vi "LS Durability Main ALTERNATE (FPGA).vi"() -> ()   [LabVIEW 2013]
uses:
  <vilib>/rvi/Emulation/niFpgaSctlEmulationGetInTimedLoop.vi
  <vilib>/rvi/Emulation/niFpgaEmulationReportErrorSimple.vi
  <vilib>/rvi/Emulation/niFpgaGetClockAttributes.vi
  <vilib>/rvi/eio/common/nirviEmuTemplateMethod_errors.vi
  <vilib>/rvi/Emulation/niFpgaCriticalErrorInLSC.vi
  <vilib>/eio/EIONode/EIONode.xnode
panel:
  out "Anomaly Resamples":fxp<+/-,28,17>[](array[numeric])
  in  "Anomaly Threshold":fxp<+/-,28,17>=0.02978515625
  out "Bank2Active":bool
  out "Bank1Active":bool
  out "Bank2On":bool
  out "Bank1On":bool
  in  "Enable Readings":bool[](array[boolean])=[FALSE, FALSE, FALSE, FALSE, FALSE, FALSE, FALSE, FALSE, FALSE, FALSE, FALSE, FALSE]
  in  "Opens Resets":bool[](array[boolean])=[FALSE, FALSE, FALSE, FALSE, FALSE, FALSE, FALSE, FALSE, FALSE, FALSE, FALSE, FALSE]
  in  "Enable Opens":bool[](array[boolean])=[FALSE, FALSE, FALSE, FALSE, FALSE, FALSE, FALSE, FALSE, FALSE, FALSE, FALSE, FALSE]
  out "Opens Detected":u16[](array[numeric])
  out "Opens Loop Time (usec)":u32=1000
  in  "Bank2(Pulse/Const)":bool
  in  "Bank2Const(On/Off)":bool
  out "Anomalies (Last Cycle)":i32[](array[numeric])
  out "Cycle Starts":bool[](array[boolean])
  out "Anomalies (Total)":i32[](array[numeric])
  out "Anomalies/Cycle":i32[](array[numeric])
  in  "Normal Steps":u32=98
  out "Cycles":u32[](array[numeric])
  out "Anomaly Loop Time (usec)":u32=1000
  out "Steps":u32[](array[numeric])
  in  "Step Threshold":fxp<+/-,28,17>=0.02978515625
  in  "Enable Anomalies":bool[](array[boolean])=[FALSE, FALSE, FALSE, FALSE, FALSE, FALSE, FALSE, FALSE, FALSE, FALSE, FALSE, FALSE]
  in  "Anomaly Resets":bool[](array[boolean])=[FALSE, FALSE, FALSE, FALSE, FALSE, FALSE, FALSE, FALSE, FALSE, FALSE, FALSE, FALSE]
  in  "Bank1Const(On/Off)":bool
  in  "Bank1(Pulse/Const)":bool
  in  "PWM Period (Ticks)":u32=4000000
  in  "Duty (Ticks)":i32=2000000
  in  "Invert PWM?":bool=TRUE
  in  "Cycle Resets":bool[](array[boolean])=[FALSE, FALSE, FALSE, FALSE, FALSE, FALSE, FALSE, FALSE, FALSE, FALSE, FALSE, FALSE]
  in  "Points to Avg":i32=20
  in  "Enable Cycles":bool[](array[boolean])=[FALSE, FALSE, FALSE, FALSE, FALSE, FALSE, FALSE, FALSE, FALSE, FALSE, FALSE, FALSE]
  out "Total Cycles":u32[](array[numeric])
  in  "Cycle Threshold":fxp<+/-,28,17>=1.2001953125
  out "AI Avg Loop Time (usec)":u32=1000
  out "Analog Inputs":fxp<+/-,28,17>[](array[numeric])
  out "AI Loop Time (usec)":u32=70
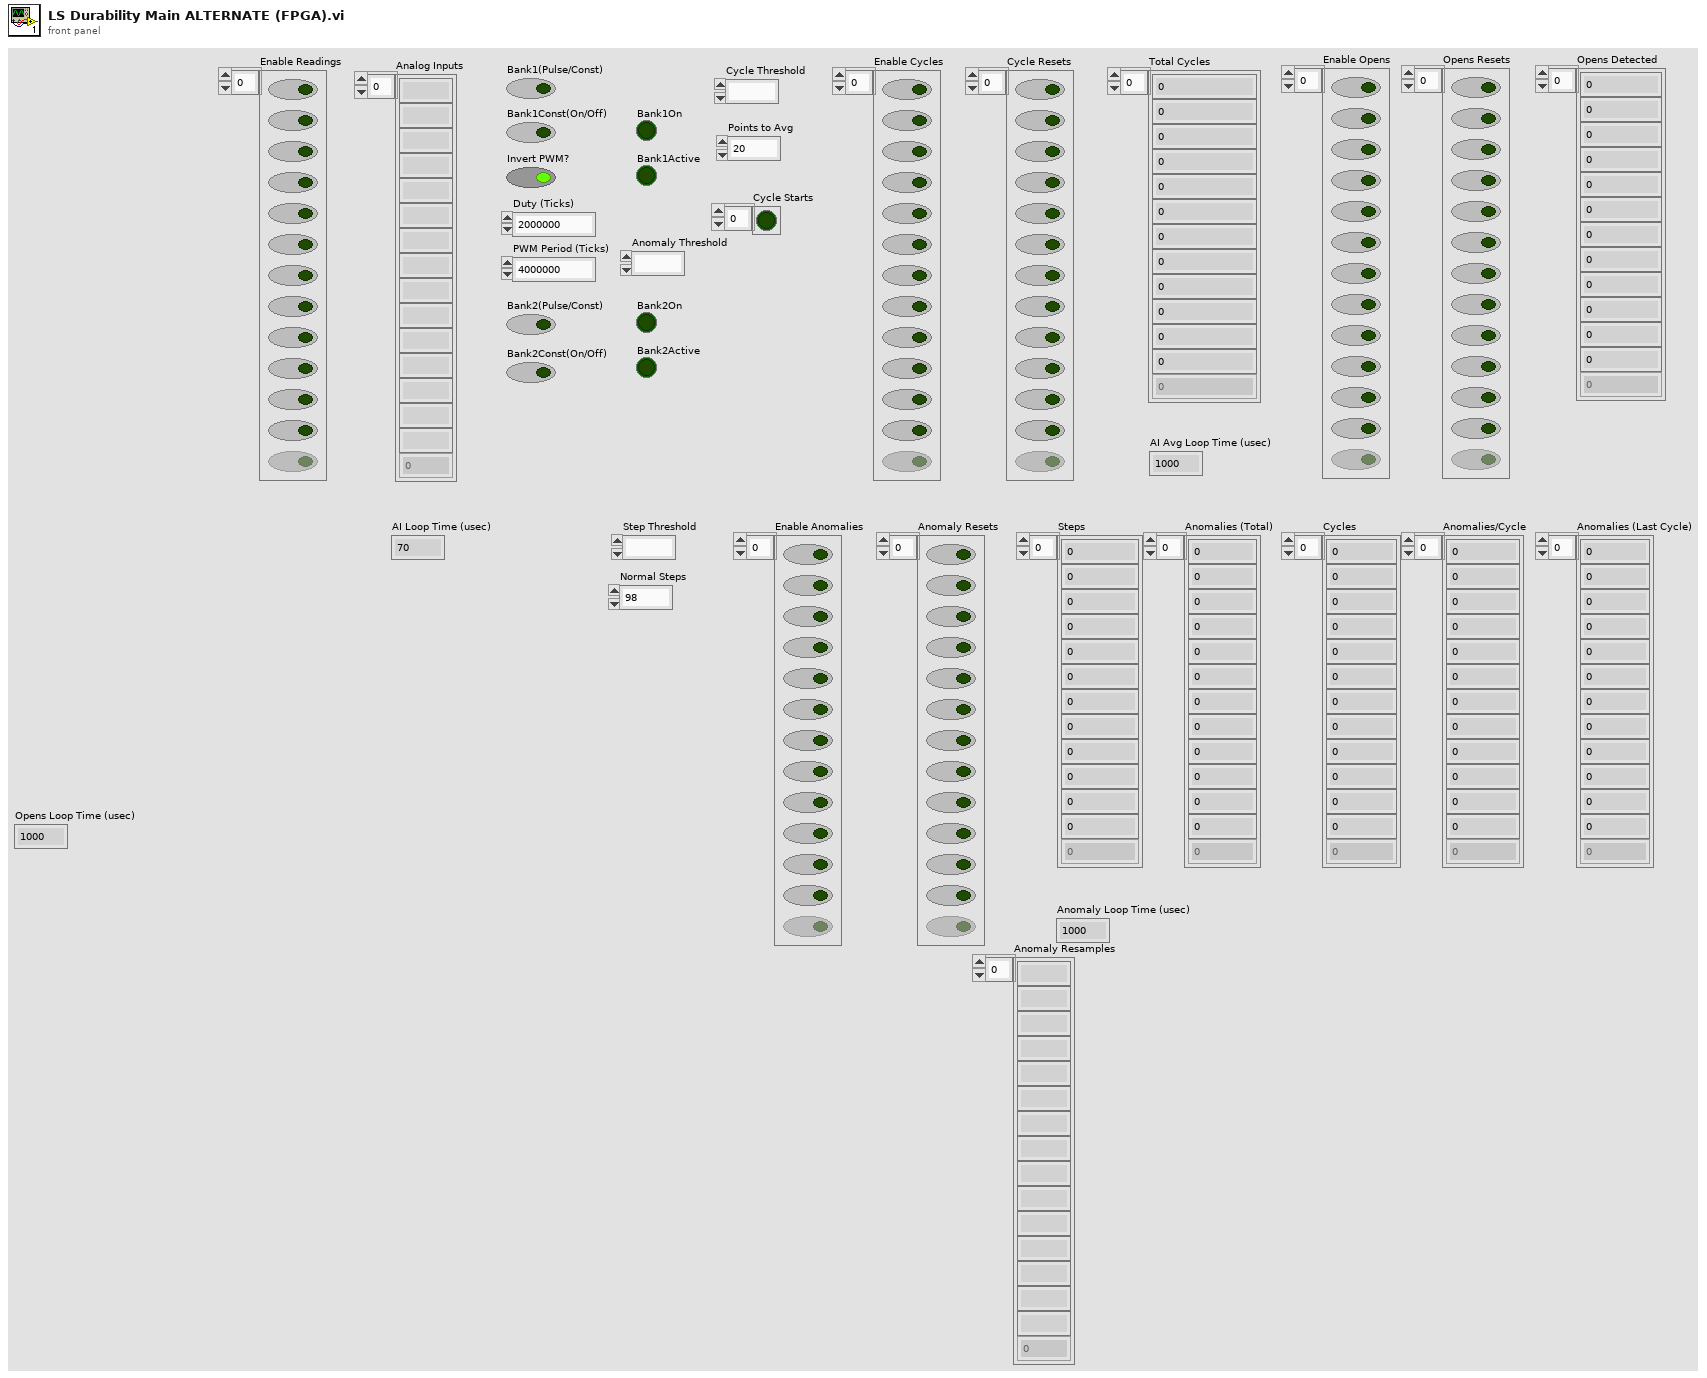
[diagram p1: front panel]
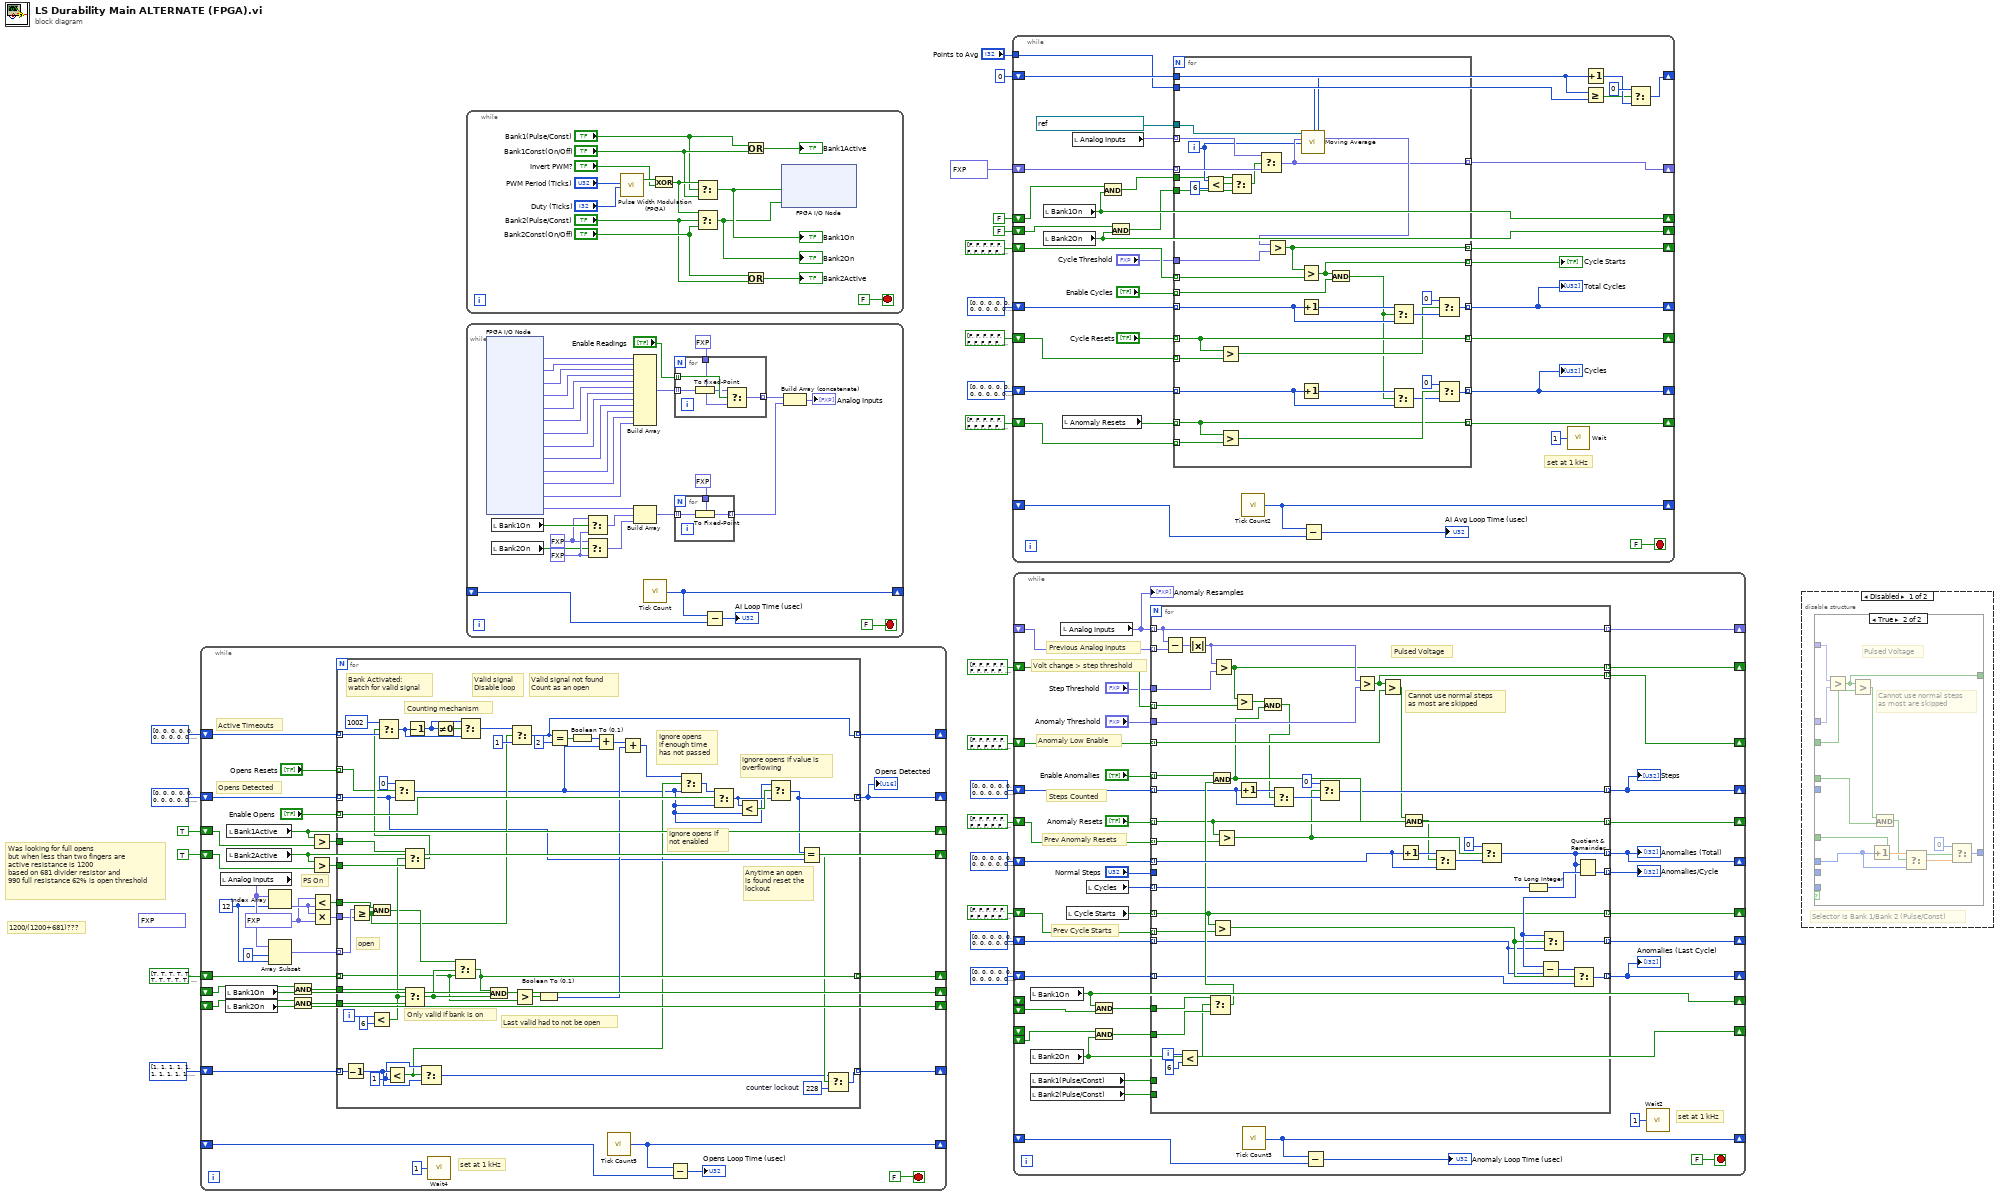
[diagram p0: block diagram]
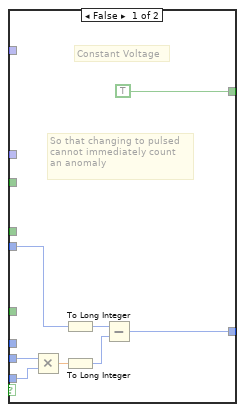
[diagram p2: hidden frame]
diagram:
  (unwired) fxp<+,8,0> 0.94921875
  # "1200/(1200+681)???"
  # "Was looking for full opens\nbut when less than two fingers are\nactive resistance is 1200\nbased on 681 divider resistor and\n990 full resistance 62% is open threshold"
  n1 = while {
    shift-right: [w57] -> _
    shift-left: _ -> [w56]
    shift-right: [w27] -> _
    shift-left: u8[] [0, 0, 0, 0, 0, 0, 0, 0, 0, 0, 0, 0] -> [w51]
    shift-right: [w36] -> _
    shift-left: u16[] [0, 0, 0, 0, 0, 0, 0, 0, 0, 0, 0, 0] -> [w37]
    shift-right: [w43] -> _
    shift-left: bool[] [TRUE, TRUE, TRUE, TRUE, TRUE, TRUE, TRUE, TRUE, TRUE, TRUE, TRUE, TRUE] -> [w42]
    shift-right: [w41] -> _
    shift-left: TRUE ("Bank2Active") -> [w39]
    shift-right: [w40] -> _
    shift-left: TRUE ("Bank1Active") -> [w38]
    shift-right: [w30] -> _
    shift-left: _ -> [w28]
    shift-right: [w31] -> _
    shift-left: _ -> [w29]
    shift-right: [w25] -> _
    shift-left: u16[] [1, 1, 1, 1, 1, 1, 1, 1, 1, 1, 1, 1] -> [w26]
    stop <- FALSE stop-if-true
    w44 = fxp<+,8,0> 0.62109375
    w53 = 12 ("length")
    # "Opens Detected"
    # "Active Timeouts"
    # "PS On"
    # "set at 1 kHz"
    n2 = local read "Analog Inputs"() -> (w54:fxp<+/-,28,17>[])
    n3 = local read "Bank1On"() -> (w31:bool)
    n4 = local read "Bank2On"() -> (w30:bool)
    n5 = local read "Bank1Active"() -> (w40:bool)
    n6 = local read "Bank2Active"() -> (w41:bool)
    n7 = Index Array(array=w54, index=w53) -> (element=w45:fxp<+/-,28,17>)
    n8 = Array Subset(array=w54, index=0, length=w53) -> (w46:fxp<+/-,28,17>[])
    n9 = And(x=w29, y=w31) -> (x .and. y?=w33:bool)
    n10 = And(x=w28, y=w30) -> (x .and. y?=w32:bool)
    n11 = Greater?(x=w40, y=w38) -> (0:w50:bool)
    n12 = Greater?(x=w41, y=w39) -> (0:w49:bool)
    n13 = Less?(x=w44, y=w45) -> (x < y?=w48:bool)
    n14 = Multiply(x=w45, y=w44) -> (x*y=w47:fxp<+/-,36,17>)
    n15 = for {
      tunnel: w33 -> [w106]
      tunnel: w32 -> [w105]
      tunnel: w50 -> [w103]
      tunnel: w49 -> [w104]
      tunnel: w51 -> [w64] mode=indexing
      tunnel: w37 -> [w91] mode=indexing
      tunnel: "Opens Resets" -> [w75] mode=indexing
      tunnel: "Enable Opens" -> [w89] mode=indexing
      tunnel: [w65] -> w27 mode=indexing
      tunnel: w47 -> [w86]
      tunnel: w46 -> [w87] mode=indexing
      tunnel: w48 -> [w85]
      tunnel: [w76] -> w43 mode=indexing
      tunnel: w42 -> [w81] mode=indexing
      tunnel: [w79] -> w36 mode=indexing
      tunnel: w26 -> [w70] mode=indexing
      tunnel: [w66] -> w25 mode=indexing
      i -> [w108]
      w67 = u16 228  # counter lockout
      w71 = u16 1 ("y")
      # "Ignore opens if\nnot enabled"
      # "Ignore opens\nif enough time\nhas not passed"
      # "Anytime an open\nis found reset the\nlockout"
      # "ignore opens if value is\noverflowing"
      # "Last valid had to not be open"
      # "Only valid if bank is on"
      # "open"
      # "Valid signal not found\nCount as an open"
      # "Valid signal\nDisable loop"
      # "Counting mechanism"
      # "Bank Activated:\nwatch for valid signal"
      n16 = Decrement(x=w70) -> (x-1=w72:u16)
      n17 = Greater Or Equal?(x=w87, y=w86) -> (x >= y?=w78:bool)
      n18 = Less?(x=w108, y=6) -> (x < y?=w102:bool)
      n19 = And(x=w85, y=w78) -> (x .and. y?=w84:bool)
      n20 = Less?(x=w72, y=w71) -> (x < y?=w61:bool)
      n21 = Select(t=u16 0, s=w75, f=w64) -> (s? t:f=w60:u16)
      n22 = Select(t=w103, s=w102, f=w104) -> (s? t:f=w88:bool)
      n23 = Select(t=u16 1002, s=w88, f=w91) -> (s? t:f=w90:u16)
      n24 = Select(t=w106, s=w102, f=w105) -> (s? t:f=w83:bool)
      n25 = Decrement(x=w90) -> (x-1=w95:u16)
      n26 = Select(t=w71, s=w61, f=w72) -> (s? t:f=w68:u16)
      n27 = Not Equal To 0?(x=w95) -> (x != 0?=w94:bool)
      n28 = Select(t=w84, s=w83, f=w81) -> (s? t:f=w76:bool)
      n29 = Select(t=w95, s=w94, f=w90) -> (s? t:f=w96:u16)
      n30 = And(x=w76, y=w83) -> (x .and. y?=w77:bool)
      n31 = Select(t=w96, s=w78, f=u16 1) -> (s? t:f=w79:u16)
      n32 = Greater?(x=w77, y=w81) -> (0:w82:bool)
      n33 = Boolean To (0,1)(Boolean=w82) -> (0, 1=w80:i16)
      n34 = Equal?(x=w79, y=u16 2) -> (x = y?=w98:bool)
      n35 = Boolean To (0,1)(Boolean=w98) -> (0, 1=w99:i16)
      n36 = Add(x=w99, y=w60) -> (x+y=w100:u16)
      n37 = Add(x=w100, y=w80) -> (x+y=w62:u16)
      n38 = Select(t=w62, s=w61, f=w60) -> (s? t:f=w63:u16)
      n39 = Select(t=w63, s=w89, f=w60) -> (s? t:f=w73:u16)
      n40 = Less?(x=w73, y=w60) -> (x < y?=w74:bool)
      n41 = Select(t=w60, s=w74, f=w73) -> (s? t:f=w65:u16)
      n42 = Equal?(x=w65, y=w64) -> (x = y?=w69:bool)
      n43 = Select(t=w68, s=w69, f=w67) -> (s? t:f=w66:u16)
    }
    "Opens Detected" <- w27
    n44 = call "Wait4"("Count(mSec)"=u32 1) -> ()  [unwired: 1 out]
    n45 = call "Tick Count5"() -> ("Tick Count(uSec)"=w57:u32)
    n46 = Subtract(x=w57, y=w56) -> (x-y=→"Opens Loop Time (usec)":u32)
  }
  n47 = while {
    shift-right: [w138] -> _
    shift-left: _ -> [w137]
    stop <- FALSE stop-if-true
    w111 = fxp<+/-,24,5> 1.0 ("AI13")
    w114 = fxp<+/-,24,5> 0.0 ("AI13")
    n48 = xnode "FPGA I/O Node"() -> ("AI0"=w135:fxp<+/-,24,5>, "AI1"=w134:fxp<+/-,24,5>, "AI2"=w133:fxp<+/-,24,5>, "AI3"=w132:fxp<+/-,24,5>, "AI4"=w131:fxp<+/-,24,5>, "AI5"=w130:fxp<+/-,24,5>, "AI6"=w129:fxp<+/-,24,5>, "AI7"=w128:fxp<+/-,24,5>, "AI8"=w127:fxp<+/-,24,5>, "AI9"=w126:fxp<+/-,24,5>, "AI10"=w125:fxp<+/-,24,5>, "AI11"=w124:fxp<+/-,24,5>, "AI12"=w121:fxp<+/-,24,5>)  [unwired: 13 in, 13 out]
    n49 = local read "Bank1On"() -> (w113:bool)
    n50 = local read "Bank2On"() -> (w112:bool)
    n51 = Select(t=w111, s=w113, f=w114) -> (s? t:f=w110:fxp<+/-,24,5>)
    n52 = Select(t=w111, s=w112, f=w114) -> (s? t:f=w109:fxp<+/-,24,5>)
    n53 = Build Array(w135, w134, w133, w132, w131, w130, w129, w128, w127, w126, w125, w124) -> (w123:fxp<+/-,24,5>[])
    n54 = Build Array(w121, w110, w109) -> (w119:fxp<+/-,24,5>[])
    n55 = call "Tick Count"() -> ("Tick Count(uSec)"=w138:u32)
    n56 = for {
      tunnel: w123 -> [w147] mode=indexing
      tunnel: fxp<+/-,28,17> 0.0 ("AI0") -> [w144]
      tunnel: [w143] -> w117 mode=indexing
      tunnel: "Enable Readings" -> [w146] mode=indexing
      n57 = To Fixed-Point(fixed-point type=w144, number=w147) -> (fixed-point=w145:fxp<+/-,28,17>)
      n58 = Select(t=w145, s=w146, f=w144) -> (s? t:f=w143:fxp<+/-,28,17>)
    }
    n59 = for {
      tunnel: w119 -> [w142] mode=indexing
      tunnel: fxp<+/-,28,17> 0.0 ("AI0") -> [w141]
      tunnel: [w140] -> w118 mode=indexing
      n60 = To Fixed-Point(fixed-point type=w141, number=w142) -> (fixed-point=w140:fxp<+/-,28,17>)
    }
    n61 = Subtract(x=w138, y=w137) -> (x-y=→"AI Loop Time (usec)":u32)
    n62 = Build Array (concatenate)(w117, w118) -> (→"Analog Inputs":fxp<+/-,28,17>[])
  }
  n63 = while {
    stop <- FALSE stop-if-true
    n64 = call "Pulse Width Modulation (FPGA).vi"("PWM Period (Ticks)"="PWM Period (Ticks)", "PWM Duty Cycle (Ticks)"="Duty (Ticks)") -> ("PWM DO"=w158:bool)  [unwired: 14 in, 3 out]
    n65 = Exclusive Or(1:"Invert PWM?", 2:w158) -> (0:w156:bool)
    n66 = Select(t=w156, s="Bank1(Pulse/Const)", f="Bank1Const(On/Off)") -> (s? t:f=w155:bool)
    "Bank1On" <- w155
    n67 = Select(t=w156, s="Bank2(Pulse/Const)", f="Bank2Const(On/Off)") -> (s? t:f=w154:bool)
    "Bank2On" <- w154
    n68 = Or(x="Bank1(Pulse/Const)", y="Bank1Const(On/Off)") -> (x .or. y?=→"Bank1Active":bool)
    n69 = Or(x="Bank2Const(On/Off)", y="Bank2(Pulse/Const)") -> (x .or. y?=→"Bank2Active":bool)
    n70 = xnode "FPGA I/O Node"("RMC/DIO0"=w155, "RMC/DIO1"=w154) -> ()  [unwired: 3 in, 3 out]
  }
  n71 = while {
    shift-right: [w191] -> _
    shift-left: 0 ("Moving Point Index") -> [w192]
    shift-right: [w187] -> _
    shift-left: _ -> [w186]
    shift-right: [w185] -> _
    shift-left: bool[] [FALSE, FALSE, FALSE, FALSE, FALSE, FALSE, FALSE, FALSE, FALSE, FALSE, FALSE, FALSE] -> [w184]
    shift-right: [w182] -> _
    shift-left: u32[] [0, 0, 0, 0, 0, 0, 0, 0, 0, 0, 0, 0] -> [w183]
    tunnel: "Points to Avg" -> [w179]
    shift-right: [w177] -> _
    shift-left: bool[] [FALSE, FALSE, FALSE, FALSE, FALSE, FALSE, FALSE, FALSE, FALSE, FALSE, FALSE, FALSE] -> [w176]
    shift-right: [w171] -> _
    shift-left: u32[] [0, 0, 0, 0, 0, 0, 0, 0, 0, 0, 0, 0] -> [w173]
    shift-right: [w174] -> _
    shift-left: bool[] [FALSE, FALSE, FALSE, FALSE, FALSE, FALSE, FALSE, FALSE, FALSE, FALSE, FALSE, FALSE] -> [w175]
    shift-right: [w167] -> _
    shift-left: FALSE -> [w165]
    shift-right: [w163] -> _
    shift-left: FALSE -> [w164]
    shift-right: [w168] -> _
    shift-left: fxp<+/-,28,17>[] [0.0, 0.0, 0.0, 0.0, 0.0, 0.0, 0.0, 0.0, 0.0, 0.0, 0.0, 0.0] ("Analog Inputs") -> [w169]
    stop <- FALSE stop-if-true
    # "set at 1 kHz"
    n72 = local read "Bank1On"() -> (w167:bool)
    n73 = local read "Bank2On"() -> (w163:bool)
    n74 = local read "Anomaly Resets"() -> (w172:bool[])
    n75 = local read "Analog Inputs"() -> (w189:fxp<+/-,28,17>[])
    n76 = And(x=w165, y=w167) -> (x .and. y?=w166:bool)
    n77 = And(x=w164, y=w163) -> (x .and. y?=w162:bool)
    n78 = for {
      tunnel: w192 -> [w230]
      tunnel: w179 -> [w231]
      tunnel: w189 -> [w206] mode=indexing
      tunnel: refnum<k21> "Running Avg Memory" ("Memory") -> [w232]
      tunnel: [w229] -> w185 mode=indexing
      tunnel: w184 -> [w228] mode=indexing
      tunnel: w183 -> [w226] mode=indexing
      tunnel: [w218] -> w182 mode=indexing
      tunnel: "Cycle Threshold" -> [w225]
      tunnel: "Enable Cycles" -> [w224] mode=indexing
      tunnel: "Cycle Resets" -> [w223] mode=indexing
      tunnel: [w223] -> w177 mode=indexing
      tunnel: w176 -> [w222] mode=indexing
      tunnel: w173 -> [w211] mode=indexing
      tunnel: [w217] -> w171 mode=indexing
      tunnel: w172 -> [w212] mode=indexing
      tunnel: [w212] -> w174 mode=indexing
      tunnel: w175 -> [w213] mode=indexing
      tunnel: [w209] -> w170 mode=indexing
      tunnel: w169 -> [w207] mode=indexing
      tunnel: [w205] -> w168 mode=indexing
      tunnel: w166 -> [w200]
      tunnel: w162 -> [w199]
      i -> [w202]
      n79 = Less?(x=w202, y=6) -> (x < y?=w203:bool)
      n80 = Greater?(x=w223, y=w222) -> (0:w220:bool)
      n81 = Greater?(x=w212, y=w213) -> (0:w215:bool)
      n82 = Select(t=w200, s=w203, f=w199) -> (s? t:f=w201:bool)
      n83 = Select(t=w206, s=w201, f=w207) -> (s? t:f=w205:fxp<+/-,28,17>)
      n84 = Increment(x=w226) -> (x+1=w227:u32)
      n85 = Increment(x=w211) -> (x+1=w210:u32)
      n86 = call "Moving Average.vi"("Memory In"=w232, "N (# of Ave Pts 127 max)"=w231, "Moving Point Index"=w230, "Data IN"=w205, "Channel#"=w202) -> ("Averaged Data"=w208:fxp<+/-,28,17>)  [unwired: 10 in]
      n87 = Greater?(x=w208, y=w225) -> (0:w229:bool)
      n88 = Greater?(x=w229, y=w228) -> (0:w209:bool)
      n89 = And(x=w209, y=w224) -> (x .and. y?=w198:bool)
      n90 = Select(t=w227, s=w198, f=w226) -> (s? t:f=w221:u32)
      n91 = Select(t=w210, s=w198, f=w211) -> (s? t:f=w214:u32)
      n92 = Select(t=u32 0, s=w220, f=w221) -> (s? t:f=w218:u32)
      n93 = Select(t=u32 0, s=w215, f=w214) -> (s? t:f=w217:u32)
    }
    "Total Cycles" <- w182
    "Cycles" <- w171
    "Cycle Starts" <- w170
    n94 = call "Tick Count2"() -> ("Tick Count(uSec)"=w187:u32)
    n95 = Subtract(x=w187, y=w186) -> (x-y=→"AI Avg Loop Time (usec)":u32)
    n96 = call "Wait"("Count(mSec)"=u32 1) -> ()  [unwired: 1 out]
    n97 = Increment(x=w192) -> (x+1=w194:i32)
    n98 = Greater Or Equal?(x=w192, y=w179) -> (x >= y?=w193:bool)
    n99 = Select(t=0, s=w193, f=w194) -> (s? t:f=w191:i32)
  }
  n100 = while {
    shift-right: [w269] -> _
    shift-left: _ -> [w268]
    shift-right: [w261] -> _
    shift-left: bool[] [FALSE, FALSE, FALSE, FALSE, FALSE, FALSE, FALSE, FALSE, FALSE, FALSE, FALSE, FALSE] -> [w260]
    shift-right: [w258] -> _
    shift-left: u32[] [0, 0, 0, 0, 0, 0, 0, 0, 0, 0, 0, 0] -> [w257]
    shift-right: [w256] -> _
    shift-left: bool[] [FALSE, FALSE, FALSE, FALSE, FALSE, FALSE, FALSE, FALSE, FALSE, FALSE, FALSE, FALSE] -> [w253]
    shift-right: [w263] -> _
    shift-left: _ -> [w262]
    shift-right: [w250] -> _
    shift-left: bool[] [FALSE, FALSE, FALSE, FALSE, FALSE, FALSE, FALSE, FALSE, FALSE, FALSE, FALSE, FALSE] -> [w249]
    shift-right: [w248] -> _
    shift-left: i32[] [0, 0, 0, 0, 0, 0, 0, 0, 0, 0, 0, 0] -> [w246]
    shift-right: [w247] -> _
    shift-left: i32[] [0, 0, 0, 0, 0, 0, 0, 0, 0, 0, 0, 0] -> [w245]
    shift-right: [w237] -> _
    shift-left: _ -> [_]
    shift-right: [w264] -> _
    shift-left: _ -> [_]
    shift-right: [w242] -> _
    shift-left: i32[] [0, 0, 0, 0, 0, 0, 0, 0, 0, 0, 0, 0] -> [w241]
    shift-right: [w238] -> _
    shift-left: bool[] [FALSE, FALSE, FALSE, FALSE, FALSE, FALSE, FALSE, FALSE, FALSE, FALSE, FALSE, FALSE] -> [w239]
    shift-left: _ -> [w235]
    shift-left: _ -> [w236]
    stop <- FALSE stop-if-true
    # "Anomaly Low Enable"
    # "Prev Cycle Starts"
    # "Prev Anomaly Resets"
    # "Steps Counted"
    # "Volt change > step threshold"
    # "Previous Analog Inputs"
    # "set at 1 kHz"
    n101 = local read "Bank1On"() -> (w237:bool)
    n102 = local read "Bank2On"() -> (w264:bool)
    n103 = local read "Bank1(Pulse/Const)"() -> (w244:bool)
    n104 = local read "Bank2(Pulse/Const)"() -> (w243:bool)
    n105 = local read "Analog Inputs"() -> (w233:fxp<+/-,28,17>[])
    "Anomaly Resamples" <- w233
    n106 = local read "Cycle Starts"() -> (w251:bool[])
    n107 = local read "Cycles"() -> (w252:u32[])
    n108 = And(x=w237, y=w236) -> (x .and. y?=w266:bool)
    n109 = And(x=w235, y=w264) -> (x .and. y?=w265:bool)
    n110 = for {
      tunnel: w233 -> [w310] mode=indexing
      tunnel: [w280] -> w261 mode=indexing
      tunnel: w260 -> [w289] mode=indexing
      tunnel: w257 -> [w282] mode=indexing
      tunnel: [w281] -> w258 mode=indexing
      tunnel: "Step Threshold" -> [w306]
      tunnel: "Enable Anomalies" -> [w309] mode=indexing
      tunnel: "Anomaly Resets" -> [w291] mode=indexing
      tunnel: [w291] -> w256 mode=indexing
      tunnel: w253 -> [w292] mode=indexing
      tunnel: [w310] -> w263 mode=indexing
      tunnel: w262 -> [w311] mode=indexing
      tunnel: "Normal Steps" -> [_]
      tunnel: w252 -> [w299] mode=indexing
      tunnel: [w298] -> w254 mode=indexing
      tunnel: [w300] -> w242 mode=indexing
      tunnel: w251 -> [w294] mode=indexing
      tunnel: [w294] -> w250 mode=indexing
      tunnel: w249 -> [w295] mode=indexing
      tunnel: [w297] -> w248 mode=indexing
      tunnel: w246 -> [w279] mode=indexing
      tunnel: [w296] -> w247 mode=indexing
      tunnel: w245 -> [w278] mode=indexing
      tunnel: w266 -> [w318]
      tunnel: w265 -> [w317]
      tunnel: w244 -> [_]
      tunnel: w243 -> [_]
      tunnel: w241 -> [w313] mode=indexing
      tunnel: "Anomaly Threshold" -> [w305]
      tunnel: w239 -> [w304] mode=indexing
      tunnel: [w303] -> w238 mode=indexing
      i -> [w316]
      # "Cannot use normal steps\nas most are skipped"
      # "Pulsed Voltage"
      n111 = Subtract(x=w310, y=w311) -> (x-y=w312:fxp<+/-,29,18>)
      n112 = Less?(x=w316, y=6) -> (x < y?=w314:bool)
      n113 = Absolute Value(x=w312) -> (abs(x)=w307:fxp<+,28,17>)
      n114 = Select(t=w318, s=w314, f=w317) -> (s? t:f=w308:bool)
      n115 = And(x=w309, y=w308) -> (x .and. y?=w288:bool)
      n116 = Greater?(x=w294, y=w295) -> (0:w293:bool)
      n117 = Greater?(x=w307, y=w306) -> (0:w280:bool)
      n118 = Greater?(x=w291, y=w292) -> (0:w284:bool)
      n119 = Greater?(x=w280, y=w289) -> (0:w290:bool)
      n120 = Increment(x=w282) -> (x+1=w285:u32)
      n121 = And(x=w290, y=w288) -> (x .and. y?=w283:bool)
      n122 = Select(t=w285, s=w283, f=w282) -> (s? t:f=w286:u32)
      n123 = Select(t=u32 0, s=w284, f=w286) -> (s? t:f=w281:u32)
      n124 = Greater?(x=w307, y=w305) -> (0:w303:bool)
      n125 = Greater?(x=w303, y=w304) -> (0:w273:bool)
      n126 = Increment(x=w313) -> (x+1=w275:i32)
      n127 = And(x=w273, y=w288) -> (x .and. y?=w274:bool)
      n128 = Select(t=w275, s=w274, f=w313) -> (s? t:f=w276:i32)
      n129 = Select(t=0, s=w284, f=w276) -> (s? t:f=w300:i32)
      n130 = To Long Integer(number=w299) -> (32bit integer=w301:i32)
      n131 = Subtract(x=w300, y=w279) -> (x-y=w302:i32)
      n132 = Select(t=w300, s=w293, f=w279) -> (s? t:f=w297:i32)
      n133 = Select(t=w302, s=w293, f=w278) -> (s? t:f=w296:i32)
      n134 = Quotient & Remainder(x=w300, y=w301) -> (floor(x/y)=w298:i32)  [unwired: 1 out]
    }
    "Steps" <- w258
    "Anomalies/Cycle" <- w254
    "Anomalies (Total)" <- w242
    "Anomalies (Last Cycle)" <- w247
    n135 = call "Tick Count3"() -> ("Tick Count(uSec)"=w269:u32)
    n136 = Subtract(x=w269, y=w268) -> (x-y=→"Anomaly Loop Time (usec)":u32)
    n137 = call "Wait2"("Count(mSec)"=u32 1) -> ()  [unwired: 1 out]
  }
  n138 = disable-structure shown="Disabled" {
    frame Disabled {
      # "Selector is Bank 1/Bank 2 (Pulse/Const)"
      n139 = case shown="True" {
        selector: _ -> [_ _]
        tunnel: _ -> [w326 _]
        tunnel: _ -> [w322 _]
        tunnel: [w321 w335] -> _
        tunnel: _ -> [w319 _]
        tunnel: _ -> [_ w336]
        tunnel: _ -> [_ w332]
        tunnel: _ -> [_ w333]
        tunnel: _ -> [_ w331]
        tunnel: _ -> [_ w330]
        tunnel: [TRUE w329] -> _
        tunnel: _ -> [_ w327]
        frame False {
          # "So that changing to pulsed\ncannot immediately count\nan anomaly"
          # "Constant Voltage"
          n140 = Multiply(x=w326, y=w322) -> (x*y=w325:dbl)
          n141 = To Long Integer(number=w319) -> (32bit integer=w324:i32)
          n142 = To Long Integer(number=w325) -> (32bit integer=w323:i32)
          n143 = Subtract(x=w324, y=w323) -> (x-y=w321:i32)
        }
        frame True {
          # "Cannot use normal steps\nas most are skipped"
          # "Pulsed Voltage"
          n144 = Greater?(x=w332, y=w331) -> (0:w329:bool)
          n145 = Greater?(x=w329, y=w330) -> (0:w328:bool)
          n146 = Increment(x=w336) -> (x+1=w337:dbl)
          n147 = And(x=w328, y=w333) -> (x .and. y?=w334:bool)
          n148 = Select(t=w337, s=w334, f=w336) -> (s? t:f=w338:dbl)
          n149 = Select(t=0, s=w327, f=w338) -> (s? t:f=w335:i32)
        }
      }
    }
    frame Enabled {
    }
  }
